vi "class_data.vi"() -> ()   [LabVIEW 2010, in "SignalWriterMH110203USBStepperMotor.lvclass"]
uses:
  SignalWriterMH110203USBStepperMotor.lvclass
  uSMC/Mode Control (uSMC).ctl
  uSMC/Set Parameters (uSMC).ctl
  uSMC/GoTo Control (uSMC).ctl
  uSMC/Get State Control (uSMC).ctl
panel:
  out "Profile Version":string="1.37"
  in  "StartPlus Default":T1={"Step motor ID"="0000000000000001", "SMname"="XYZ", "Backlash"=0, "wait for input sygnal to start"=FALSE, "use slow start/stop"=TRUE, "units name"="steps", "Maximum speed"=5000.0, "speed"=1500.0, "step"=3, "point 1 ticks"=0, "point 2 ticks"=64, "point 1 units"=0.0, "point 2 units"=1.0, "Limit Switch standoff"=0.0, "Zero Value"=0.0, "Destination Position"=0.0, "force backlash"=FALSE, "power off when stop"=FALSE, "POff delay"=600.0, "positioner name"="Linear", "R, Ohm"=0.0, "I, mA"=0.0, "Positioner's Type"=0, "Reset Direction"=FALSE, "Manufacturer"="Unknown", "Model"="Unknown", "Scheme"="4Wire", "FirmwareVer"="unknown"} {"Positioner's Type" items=["Linear", "Rotational"]; "POff delay" min=1.0}
  out "Position Default":T2={"Cur Pos Units"=0.0, "Set Cur Pos units"=0.0, "Lo Limit Units"=-33554428.0, "Hi Limit Units"=33554427.78, "Cur Pos Ticks"=0, "Set Cur Pos ticks"=0, "Lo Limit Ticks"=-2147483648, "Hi Limit Ticks"=2147483647, "Minimal Value"=-33554428.0, "Maximal Value"=33554427.78} {"Hi Limit Units" format="%#.6f"; "Lo Limit Units" format="%#.6f"}
  out "Parameters Defalut":T3={"Acceleration Time"=38, "Deceleration Time"=38, "Reduce Current Timeout"=1000, "Buttons Timeout 1"=500, "Buttons Timeout 2"=1000, "Buttons Timeout 3"=1500, "Buttons Timeout 4"=2000, "Buttons Timeout Reset"=2000, "Buttons Timeout DblClick"=294, "Reset Speed"=64, "Buttons Speed 1"=3, "Buttons Speed 2"=13, "Buttons Speed 3"=32, "Buttons Speed 4"=64, "Max Backlash"=1024, "Start Pos"=0, "RTdelta"=200, "RTMinError"=5, "Maximum Temperature"=24872, "Sync Duration"=5, "Backlash Speed"=3, "EncVSCP"=10, "Steps Per Revolution"=0, "Encoder Pulses Per Rev-on"=0}
  out "Mode Defalults":T4={"Turn Buttons Off"=FALSE, "Reduce Current"=TRUE, "Power Off and Make a Whole Step"=TRUE, "Emergency Power Off"=FALSE, "Limit Switch 1 True State"=FALSE, "Limit Switch 2 True State"=FALSE, "Rotary Transducer TRUE State"=TRUE, "Swap Limit Switches"=TRUE, "Limit Switch 1 Operation Enabled"=TRUE, "Limit Switch 2 Operation Enabled"=TRUE, "Rotary Transducer Operation Enabled"=FALSE, "Rotary Transducer Operation Select"=TRUE, "Button 1 True State"=FALSE, "Button 2 True State"=FALSE, "Swap Buttons"=FALSE, "Reset Rotary Transducer Check Positions"=TRUE, "Output Syncronization Enabled"=FALSE, "Reset Output Sync Count"=FALSE, "Sync Operation"=FALSE, "Sync Count"=50, "Power"=TRUE, "Invert Sync Polarity"=FALSE, "Use Encoder"=FALSE, "Invert Encoder Direction"=FALSE, "Reset Encoder To 0"=FALSE, "Reset SM Enc Pos to Enc Pos"=FALSE}
  out "Current State":T5[](array[typedef])
  in  "StartPlus Array":T1[](array[typedef]) {"Positioner's Type" items=["Linear", "Rotational"]; "POff delay" min=1.0}
  out "Position Array":T6(array[cluster]) {"Hi Limit Units" format="%#.6f"; "Lo Limit Units" format="%#.6f"}
  out "Parameters Array":T3[](array[typedef])
  out "Mode Array":T4[](array[typedef])
  out "Firmware Versions":string[](array[string])
  # "RUN-TIME PARAMETERS"
  # "DEFAULT PARAMETERS"
  # "all time is in ms\nall speed is in Full Steps/sec"
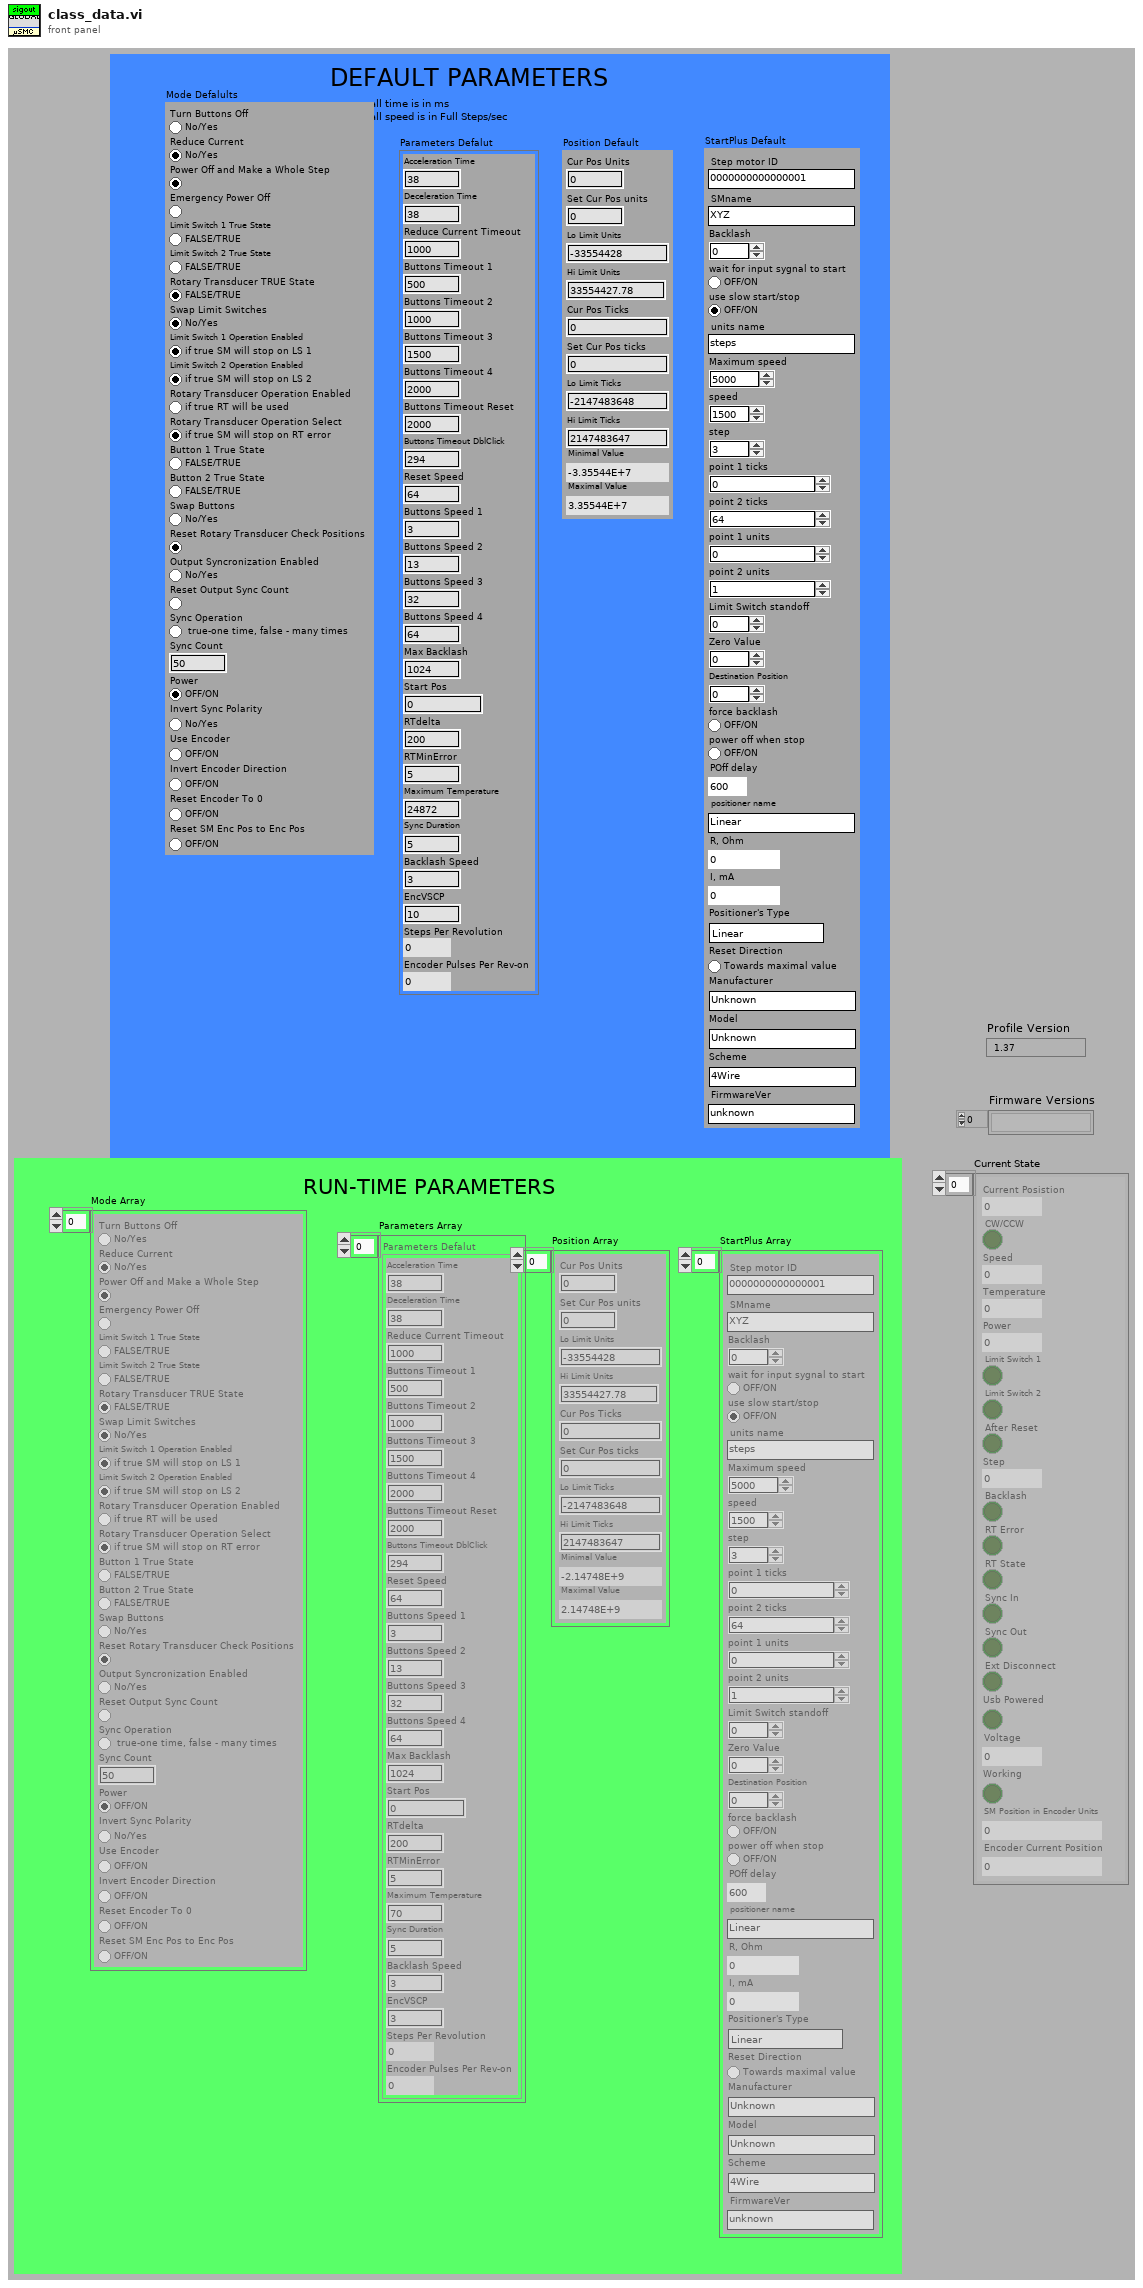
[diagram p1: front panel]
types:
  T1 = typedef "SignalWriterMH110203USBStepperMotor.lvclass/GoTo Control (uSMC).ctl" = cluster{"Step motor ID":string, "SMname":string, "Backlash":u16, "wait for input sygnal to start":bool, "use slow start/stop":bool, "units name":string, "Maximum speed":dbl, "speed":dbl, "step":u8, "point 1 ticks":i32, "point 2 ticks":i32, "point 1 units":dbl, "point 2 units":dbl, "Limit Switch standoff":dbl, "Zero Value":dbl, "Destination Position":dbl, "force backlash":bool, "power off when stop":bool, "POff delay":dbl, "positioner name":string, "R, Ohm":dbl, "I, mA":dbl, "Positioner's Type":u16, "Reset Direction":bool, "Manufacturer":string, "Model":string, "Scheme":string, "FirmwareVer":string}
  T2 = cluster{"Cur Pos Units":dbl, "Set Cur Pos units":dbl, "Lo Limit Units":dbl, "Hi Limit Units":dbl, "Cur Pos Ticks":i32, "Set Cur Pos ticks":i32, "Lo Limit Ticks":i32, "Hi Limit Ticks":i32, "Minimal Value":dbl, "Maximal Value":dbl}
  T3 = typedef "SignalWriterMH110203USBStepperMotor.lvclass/Set Parameters (uSMC).ctl" = cluster{"Acceleration Time":u8, "Deceleration Time":u8, "Reduce Current Timeout":u16, "Buttons Timeout 1":u16, "Buttons Timeout 2":u16, "Buttons Timeout 3":u16, "Buttons Timeout 4":u16, "Buttons Timeout Reset":u16, "Buttons Timeout DblClick":u16, "Reset Speed":u16, "Buttons Speed 1":u16, "Buttons Speed 2":u16, "Buttons Speed 3":u16, "Buttons Speed 4":u16, "Max Backlash":u16, "Start Pos":i32, "RTdelta":u16, "RTMinError":u16, "Maximum Temperature":u16, "Sync Duration":u8, "Backlash Speed":u16, "EncVSCP":u8, "Steps Per Revolution":i32, "Encoder Pulses Per Rev-on":i32}
  T4 = typedef "SignalWriterMH110203USBStepperMotor.lvclass/Mode Control (uSMC).ctl" = cluster{"Turn Buttons Off":bool, "Reduce Current":bool, "Power Off and Make a Whole Step":bool, "Emergency Power Off":bool, "Limit Switch 1 True State":bool, "Limit Switch 2 True State":bool, "Rotary Transducer TRUE State":bool, "Swap Limit Switches":bool, "Limit Switch 1 Operation Enabled":bool, "Limit Switch 2 Operation Enabled":bool, "Rotary Transducer Operation Enabled":bool, "Rotary Transducer Operation Select":bool, "Button 1 True State":bool, "Button 2 True State":bool, "Swap Buttons":bool, "Reset Rotary Transducer Check Positions":bool, "Output Syncronization Enabled":bool, "Reset Output Sync Count":bool, "Sync Operation":bool, "Sync Count":u32, "Power":bool, "Invert Sync Polarity":bool, "Use Encoder":bool, "Invert Encoder Direction":bool, "Reset Encoder To 0":bool, "Reset SM Enc Pos to Enc Pos":bool}
  T5 = typedef "SignalWriterMH110203USBStepperMotor.lvclass/Get State Control (uSMC).ctl" = cluster{"Current Posistion":dbl, "CW/CCW":bool, "Speed":u16, "Temperature":dbl, "Power":u16, "Limit Switch 1":bool, "Limit Switch 2":bool, "After Reset":bool, "Step":u8, "Backlash":bool, "RT Error":bool, "RT State":bool, "Sync In":bool, "Sync Out":bool, "Ext Disconnect":bool, "Usb Powered":bool, "Voltage":dbl, "Working":bool, "SM Position in Encoder Units":i32, "Encoder Current Position":i32}
  T6 = cluster{"Cur Pos Units":dbl, "Set Cur Pos units":dbl, "Lo Limit Units":dbl, "Hi Limit Units":dbl, "Cur Pos Ticks":i32, "Set Cur Pos ticks":i32, "Lo Limit Ticks":i32, "Hi Limit Ticks":i32, "Minimal Value":dbl, "Maximal Value":dbl}[]
diagram:
